vi "UMLEditor_PlaceVIsOnBlockDiagram.vi"(1 "BD":refnum<vi>, 2 "StartPos":cluster{i32, u32}, 3 "VIs":path[](array[path]), 5 "error in (no error)":errorcluster) -> (19 "error out":errorcluster)   [LabVIEW 2020]
doc: "Gets current diagram values"
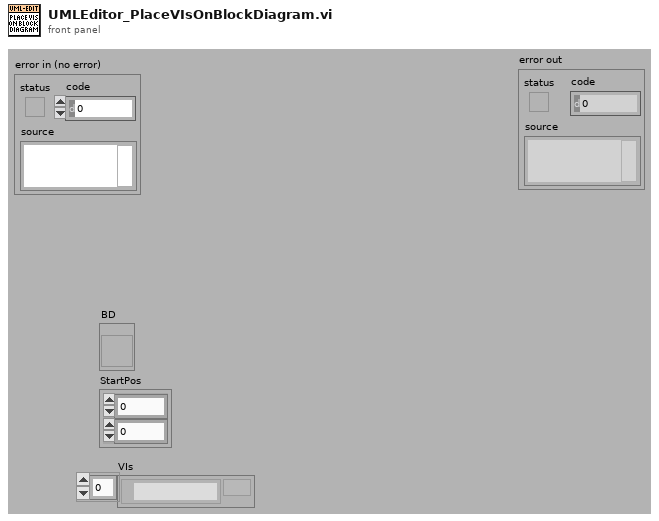
[diagram p1: front panel]
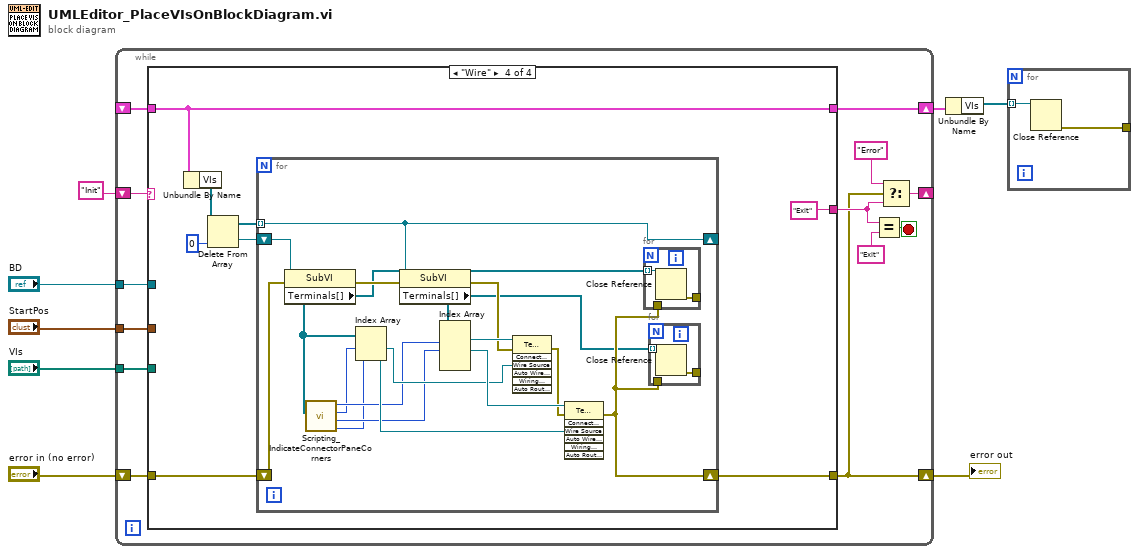
[diagram p0: block diagram]
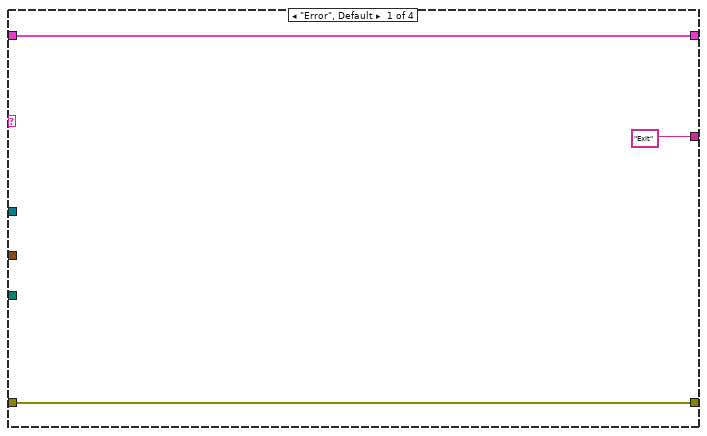
[diagram p2: hidden frame]
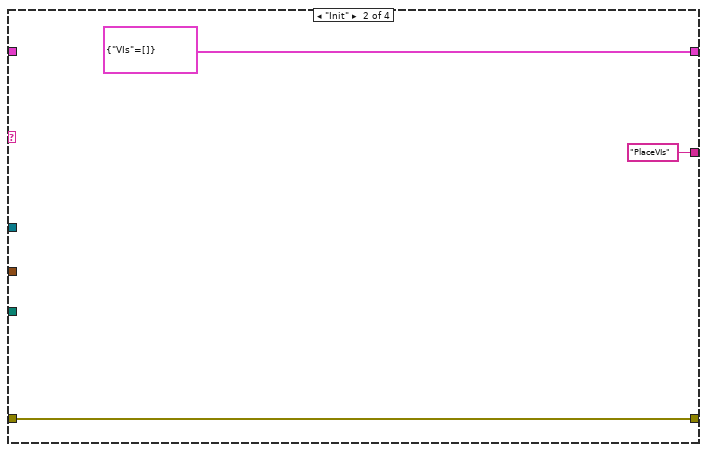
[diagram p3: hidden frame]
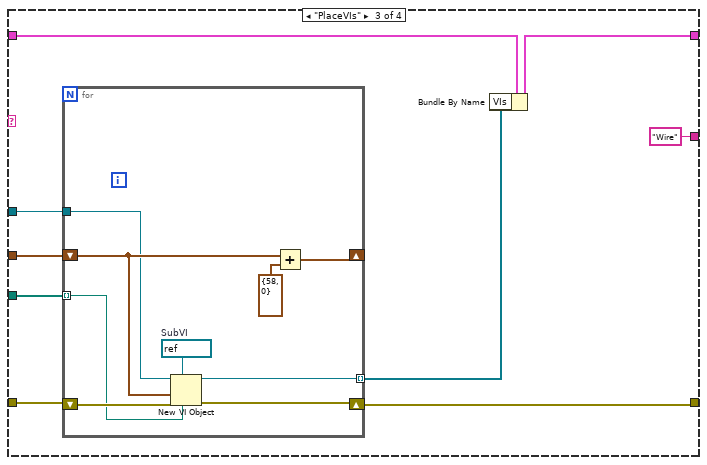
[diagram p4: hidden frame]
diagram:
  n1 = while {
    shift-right: [w14] -> w6
    shift-left: "error in (no error)" -> [w21]
    shift-right: [w19] -> _
    shift-left: "Init" -> [w20]
    shift-right: [w13] -> w2
    shift-left: _ -> [w12]
    tunnel: "VIs" -> [w11]
    tunnel: "StartPos" -> [w10]
    tunnel: "BD" -> [w9]
    stop <- w18 stop-if-true
    n2 = case shown="\"Wire\"" w20 {
      tunnel: w21 -> [w24 w27 w34 w51]
      tunnel: [w24 w27 w33 w50] -> w14
      tunnel: ["Exit" "PlaceVIs" "Wire" "Exit"] -> w15
      tunnel: [w23 cluster{"VIs":refnum<vi>[]} {"VIs"=[]} w29 w52] -> w13
      tunnel: w12 -> [w23 _ w30 w52]
      tunnel: w11 -> [_ _ w35 _]
      tunnel: w10 -> [_ _ w32 _]
      tunnel: w9 -> [_ _ w31 _]
      frame "Error", Default {
      }
      frame "Init" {
      }
      frame "PlaceVIs" {
        n3 = for {
          tunnel: w35 -> [w40] mode=indexing
          shift-right: [w39] -> w33
          shift-left: w34 -> [w45]
          shift-right: [w42] -> _
          shift-left: w32 -> [w44]
          tunnel: w31 -> [w38]
          tunnel: [w37] -> w28 mode=indexing
          w41 = refnum<vi> refnum  # SubVI
          n4 = New VI Object(vi object class=w41, owner refnum=w38, position/next to=w44, 6:w40, 8:w45) -> (object refnum=w37:refnum<vi>, 0:w39:errorcluster)  [unwired: 3 out]
          n5 = Add(x=w44, y=cluster{i32, u32} {58, 0}) -> (x+y=w42:cluster{i32, u32})
        }
        n6 = Bundle By Name(cluster=w30, "VIs"=w28) -> (w29:cluster{"VIs":refnum<vi>[]})
      }
      frame "Wire" {
        n7 = Unbundle By Name(w52) -> ("VIs"=w49:refnum<vi>[])
        n8 = Delete From Array(array=w49, index=0) -> (deleted portion=w48:refnum<vi>, array with subset deleted=w47:refnum<vi>[])  [unwired: 1 in]
        n9 = for {
          shift-right: [w60] -> w50
          shift-left: w51 -> [w69]
          shift-right: [w67] -> _
          shift-left: w48 -> [w70]
          tunnel: w47 -> [w67] mode=indexing
          n10 = property class="SubVI"(reference=w70, error in=w69) -> (error out=w68:errorcluster, "Terminals[]"=w58:refnum<vi>[])  [unwired: 1 out]
          n11 = call <resource>:"Scripting_IndicateConnectorPaneCorners.vi"("Terminals[]"=w58) -> ("RightLower"=w54:i32, "LeftLower"=w56:i32, "RightTop"=w55:i32, "LeftTop"=w57:i32)  [unwired: 1 in, 6 out]
          n12 = Index Array(array=w58, index #1=w55, index #2=w54) -> (element #1=w63:refnum<vi>, element #2=w66:refnum<vi>)
          n13 = property class="SubVI"(reference=w67, error in=w68) -> (error out=w62:errorcluster, "Terminals[]"=w59:refnum<vi>[])  [unwired: 1 out]
          n14 = Index Array(array=w59, index #1=w57, index #2=w56) -> (element #1=w64:refnum<vi>, element #2=w65:refnum<vi>)  [unwired: 2 in, 2 out]
          n15 = invoke class="Term" method="Connect Wire"(reference=w64, error in=w62, "Wire Source"=w63) -> (error out=w61:errorcluster)  [unwired: 4 in, 6 out]
          n16 = invoke class="Term" method="Connect Wire"(reference=w65, error in=w61, "Wire Source"=w66) -> (error out=w60:errorcluster)  [unwired: 4 in, 6 out]
          n17 = for {
            tunnel: w60 -> [_]
            tunnel: w58 -> [w74] mode=indexing
            tunnel: [w73] -> _
            n18 = Close Reference(reference=w74) -> (error out=w73:errorcluster)  [unwired: 1 in]
          }
          n19 = for {
            tunnel: w60 -> [_]
            tunnel: w59 -> [w72] mode=indexing
            tunnel: [w71] -> _
            n20 = Close Reference(reference=w72) -> (error out=w71:errorcluster)  [unwired: 1 in]
          }
        }
      }
    }
    n21 = Equal?(x=w15, y="Exit") -> (x = y?=w18:bool)
    n22 = Select(t="Error", s=w14, f=w15) -> (s? t:f=w19:string)
  }
  "error out" <- w6
  n23 = Unbundle By Name(w2) -> ("VIs"=w1:refnum<vi>[])
  n24 = for {
    tunnel: w1 -> [w76] mode=indexing
    tunnel: [w75] -> _
    n25 = Close Reference(reference=w76) -> (error out=w75:errorcluster)  [unwired: 1 in]
  }
